vi "CAN Frames Read.vi"(7 "Channel Number":u32, 8 "error in (no error)":errorcluster, 9 "timeout [ms]":u32=100, 11 "FPGA Refnum":T1) -> (0 "error out":errorcluster, 1 "Valid":bool, 2 "Frames":T2[](array[typedef]) {"payload" format="%x"; "timestamp" format="%<%.7X\n%x>T"; "type" items=["CAN Data"=0, "CAN Remote"=1, "CAN Bus Error"=2, "CAN 2.0 Data"=8, "CAN FD Data"=16, "CAN FD+BRS Data"=24, "J1939 Data"=192, "Delay"=224, "Log Trigger"=225, "Start Trigger"=226]; "identifier" format="%x"})   [LabVIEW 2020, in "985x Support Addon Engine.lvlib"]
uses:
  985x Support Addon Engine.lvlib
  <vilib>/xnet/xnet.llb/XNET Frame CAN.ctl
  <vilib>/xnet/xnet.llb/XNET Frame Type CAN.ctl
  Types/FPGA Refnum.ctl
  <vilib>/Utility/error.llb/Error Cluster From Error Code.vi
  <vilib>/rvi/errors/niLvFpgaAdjustHostInterfaceError.vi
  <vilib>/rvi/interface/nirviMethod/nirviMethod.xnode
  <vilib>/FPGAPlugInAG/Dynamic/niLvFpga_ReadFifo_Dynamic.vi
  <vilib>/rvi/errors/niLvFpgaMergeErrorWithErrorCode.vi
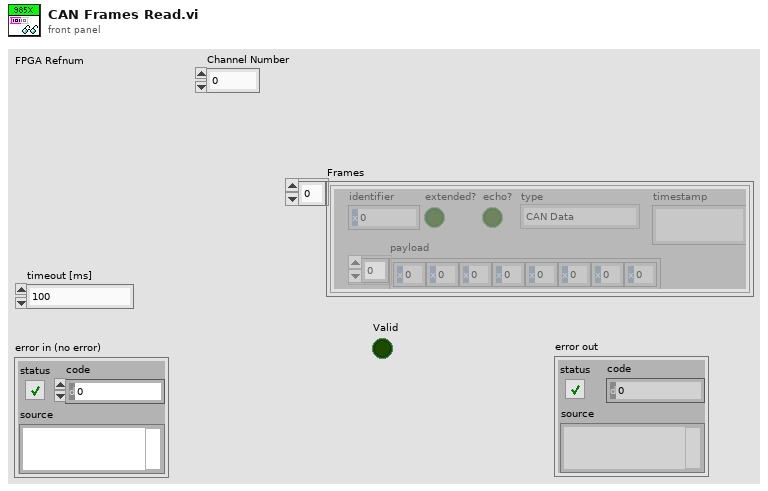
[diagram p1: front panel]
types:
  T1 = typedef "985x Support Addon Engine.lvlib/FPGA Refnum.ctl" = refnum<k20>
  T2 = typedef "XNET Frame CAN.ctl" = cluster{"timestamp":timestamp, "payload":u8[], "identifier":u32, "type":T3, "extended?":bool, "echo?":bool}
  T3 = typedef "XNET Frame Type CAN.ctl" = u8
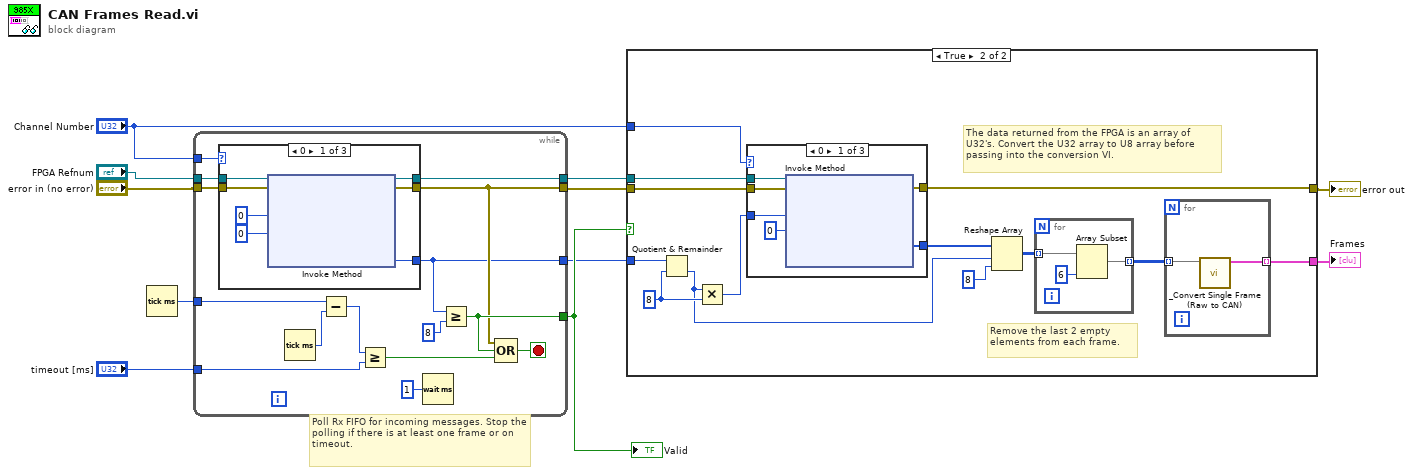
[diagram p0: block diagram]
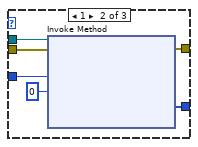
[diagram p3: hidden frame]
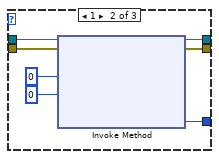
[diagram p5: hidden frame]
diagram:
  # "Poll Rx FIFO for incoming messages. Stop the polling if there is at least one frame or on timeout."
  n1 = Tick Count (ms)() -> (millisecond timer value=w11:u32)
  n2 = while {
    tunnel: "FPGA Refnum" -> [w26]
    tunnel: "error in (no error)" -> [w25]
    tunnel: w11 -> [w23]
    tunnel: "timeout [ms]" -> [w20]
    tunnel: [w18] -> w9
    tunnel: [w15] -> w7
    tunnel: [w14] -> w8
    tunnel: [w13] -> w6
    tunnel: "Channel Number" -> [w12]
    stop <- w16 stop-if-true
    n3 = case shown="0" w12 {
      tunnel: w26 -> [w33 w40 w42]
      tunnel: w25 -> [w32 w39 w41]
      tunnel: [w29 w36 w42] -> w15
      tunnel: [w28 w35 w41] -> w14
      tunnel: [w27 w34 _] -> w13
      frame 0 {
        n4 = xnode "Invoke Method"("FPGA VI Reference In"=w33, "error in"=w32, "Number of Elements"=u32 0, "Timeout (ms)"=0) -> ("FPGA VI Reference Out"=w29:T1, "error out"=w28:errorcluster, "Elements Remaining"=w27:u32)  [unwired: 1 out]
      }
      frame 1 {
        n5 = xnode "Invoke Method"("FPGA VI Reference In"=w40, "error in"=w39, "Number of Elements"=u32 0, "Timeout (ms)"=0) -> ("FPGA VI Reference Out"=w36:T1, "error out"=w35:errorcluster, "Elements Remaining"=w34:u32)  [unwired: 1 out]
      }
      frame Default {
      }
    }
    n6 = Tick Count (ms)() -> (millisecond timer value=w22:u32)
    n7 = Subtract(x=w23, y=w22) -> (x-y=w21:u32)
    n8 = Greater Or Equal?(x=w21, y=w20) -> (x >= y?=w17:bool)
    n9 = Wait (ms)(milliseconds to wait=u32 1) -> ()  [unwired: 1 out]
    n10 = Greater Or Equal?(x=w13, y=u32 8) -> (x >= y?=w18:bool)
    n11 = Compound Arithmetic op=OR(w14, w18, w17) -> (w16:bool)
  }
  "Valid" <- w9
  n12 = case shown="True" w9 {
    tunnel: [w43 w51] -> w5
    tunnel: w8 -> [w43 w54]
    tunnel: w7 -> [_ w56]
    tunnel: w6 -> [_ w55]
    tunnel: [_ w45] -> w4
    tunnel: "Channel Number" -> [_ w44]
    frame False {
    }
    frame True {
      w52 = u32 8 ("y")
      # "The data returned from the FPGA is an array of U32's. Convert the U32 array to U8 array before passing into the conversion VI."
      # "Remove the last 2 empty elements from each frame."
      n13 = Quotient & Remainder(x=w55, y=w52) -> (floor(x/y)=w47:u32)  [unwired: 1 out]
      n14 = Multiply(x=w47, y=w52) -> (x*y=w53:u32)
      n15 = case shown="0" w44 {
        tunnel: w56 -> [w62 w68 _]
        tunnel: w54 -> [w61 w67 w69]
        tunnel: w53 -> [w60 w66 _]
        tunnel: [w58 w64 w69] -> w51
        tunnel: [w57 w63 _] -> w49
        frame 0 {
          n16 = xnode "Invoke Method"("FPGA VI Reference In"=w62, "error in"=w61, "Number of Elements"=w60, "Timeout (ms)"=0) -> ("error out"=w58:errorcluster, "Data"=w57:u32[])  [unwired: 2 out]
        }
        frame 1 {
          n17 = xnode "Invoke Method"("FPGA VI Reference In"=w68, "error in"=w67, "Number of Elements"=w66, "Timeout (ms)"=0) -> ("error out"=w64:errorcluster, "Data"=w63:u32[])  [unwired: 2 out]
        }
        frame Default {
        }
      }
      n18 = Reshape Array(w49, w47, 8 ("y")) -> (w48:u32[][])
      n19 = for {
        tunnel: w48 -> [w74] mode=indexing
        tunnel: [w72] -> w46 mode=indexing
        n20 = Array Subset(array=w74, length=6) -> (w72:u32[])  [unwired: 1 in]
      }
      n21 = for {
        tunnel: w46 -> [w70] mode=indexing
        tunnel: [w71] -> w45 mode=indexing
        n22 = call "_Convert Single Frame (Raw to CAN).vi"("Raw U32"=w70) -> ("CAN frame"=w71:T2)  [unwired: 8 in, 1 out]
      }
    }
  }
  "error out" <- w5
  "Frames" <- w4
